vi "CreatePrivateEvents.vi"(8 "error in (no error)":errorcluster, 11 "Logger":refnum<class "Logger.PGSQL.lvclass">) -> (0 "error out":errorcluster, 3 "Logger out":refnum<class "Logger.PGSQL.lvclass">)   [LabVIEW 2019, in "Logger.PGSQL.lvlib" / "Logger.PGSQL.lvclass"]
doc: "---------------------------------------------------------------\nJKI State Machine Objects™\nhttp://jki.net/state-machine-objects/\nCopyright (C) 2005-2015, JKI <info@jki.net>\nALL RIGHTS RESERVEDJKI State Machine Objects (SMO) 1.0.0.4\nJKI - JKI\nCopyright (c) 2015, JKI"
uses:
  Logger.PGSQL.lvclass
  Typedefs/PrivateEvents--Logger.PGSQL.Set Address.ctl
  Typedefs/PrivateEvents--Logger.PGSQL.Write Variable.ctl
  Typedefs/PrivateEvents--Logger.PGSQL.Read Variable.ctl
  Logger.PGSQL.lvclass/Logger.PGSQL.ctl
  <userlib>/LevyLab/Logger/Logger/Logger.lvclass
panel:
  # "For instructions on how to use the JKI State Machine Objects, examples and video tutorials, visit:\nhttp://jki.net/state-machine-objects/\n\nJKI State Machine Objects™\nhttp://jki.net/state-machine-objects/\nCopyright (C) 2005-2015, JKI <info@jki.net>\nALL RIGHTS RESERVED"
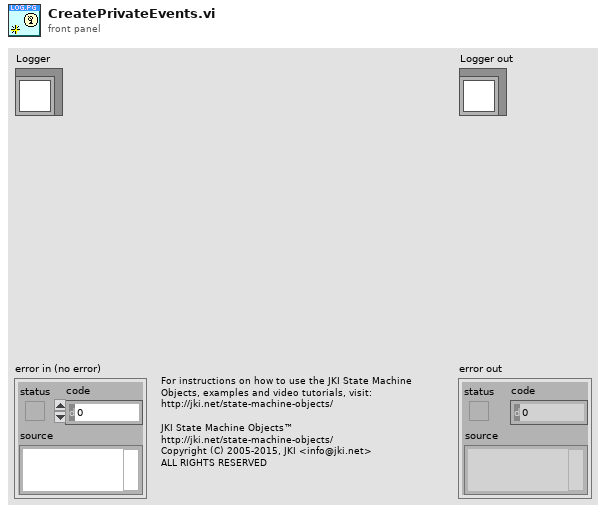
[diagram p1: front panel]
types:
  T1 = typedef "Logger.PGSQL.lvlib/Logger.PGSQL.lvclass/PrivateEvents--Logger.PGSQL.Read Variable.ctl" = cluster{"Address":string}
  T2 = typedef "Logger.PGSQL.lvlib/Logger.PGSQL.lvclass/PrivateEvents--Logger.PGSQL.Write Variable.ctl" = cluster{"Address":string, "Data":variant}
  T3 = typedef "Logger.PGSQL.lvlib/Logger.PGSQL.lvclass/PrivateEvents--Logger.PGSQL.Set Address.ctl" = string
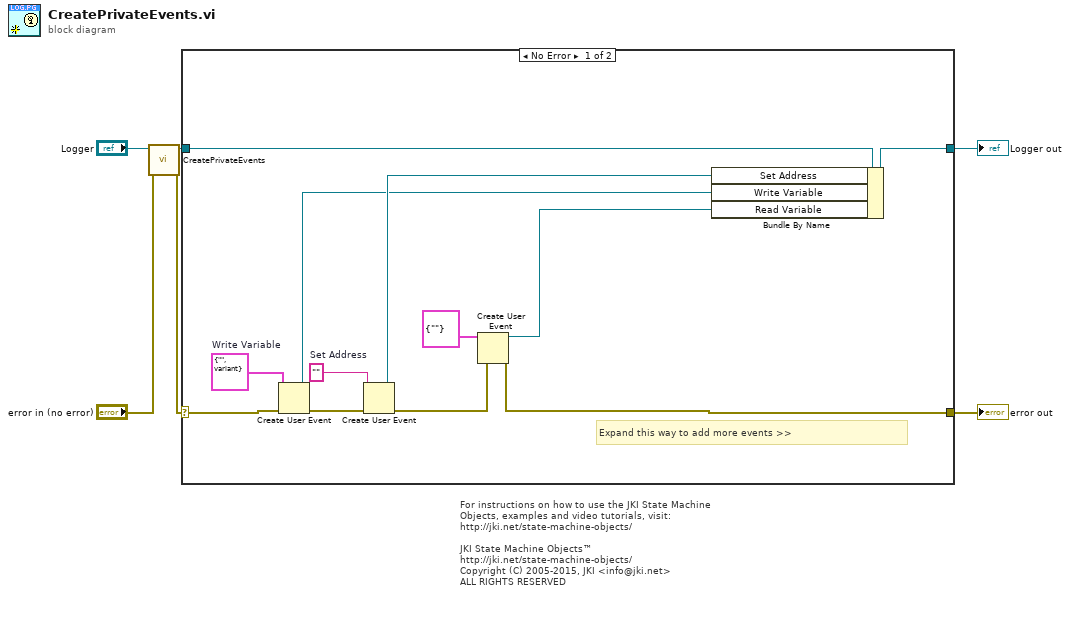
[diagram p0: block diagram]
diagram:
  # "For instructions on how to use the JKI State Machine Objects, examples and video tutorials, visit:\nhttp://jki.net/state-machine-objects/\n\nJKI State Machine Objects™\nhttp://jki.net/state-machine-objects/\nCopyright (C) 2005-2015, JKI <info@jki.net>\nALL RIGHTS RESERVED"
  n1 = call-parent "CreatePrivateEvents.vi"("error in (no error)"="error in (no error)", "SMO"="Logger") -> ("error out"=w1:errorcluster, "SMO out"=w3:refnum<class "Logger.PGSQL.lvclass">)  [unwired: 8 in]
  n2 = case shown="No Error" w1 {
    selector: w1 -> [w17 w20]
    tunnel: [w7 w20] -> w5
    tunnel: [w16 w19] -> w6
    tunnel: w3 -> [w18 w19]
    frame No Error {
      w12 = T2 {"Address"="", "Data"=variant(dbl 0.0)}  # Write Variable
      w15 = T3 ""  # Set Address
      # "Expand this way to add more events >>"
      n3 = Create User Event(user event datatype=w12, error in=w17) -> (user event=w11:refnum<user-event>, error out=w13:errorcluster)
      n4 = Create User Event(user event datatype=w15, error in=w13) -> (user event=w14:refnum<user-event>, error out=w8:errorcluster)
      n5 = Create User Event(user event datatype=T1 {"Address"=""} ("Read Variable"), error in=w8) -> (user event=w9:refnum<user-event>, error out=w7:errorcluster)
      n6 = Bundle By Name(cluster=w18, "Set Address"=w14, "Write Variable"=w11, "Read Variable"=w9) -> (w16:refnum<class "Logger.PGSQL.lvclass">)
    }
    frame Error {
    }
  }
  "error out" <- w5
  "Logger out" <- w6
